vi "HB_SumStringOfBytes.vi"(1 "String Of Bytes":string) -> (0 "Sum as String":string)   [LabVIEW 2016]
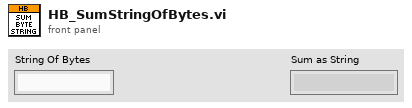
[diagram p1: front panel]
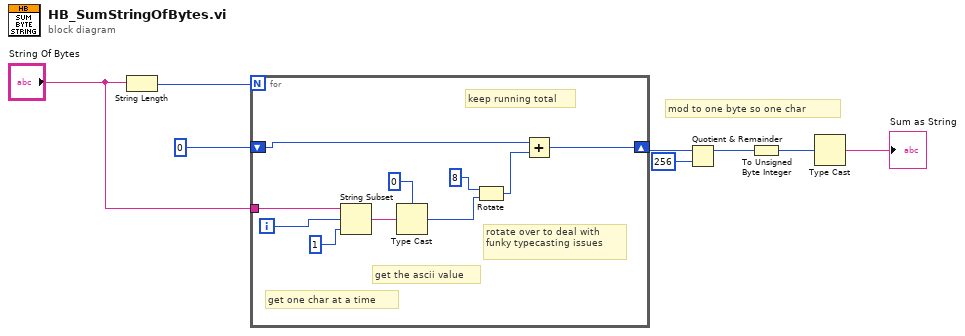
[diagram p0: block diagram]
diagram:
  # "mod to one byte so one char"
  n1 = String Length(string="String Of Bytes") -> (length=w8:i32)
  n2 = for {
    N: w8 -> [_]
    tunnel: "String Of Bytes" -> [w18]
    shift-right: [w12] -> w5
    shift-left: 0 -> [w13]
    i -> [w17]
    # "keep running total"
    # "rotate over to deal with\nfunky typecasting issues"
    # "get the ascii value"
    # "get one char at a time"
    n3 = String Subset(string=w18, offset (0)=w17, length (rest)=1 ("length (rest)")) -> (substring=w15:string)
    n4 = Type Cast(type=0 ("length (rest)"), x=w15) -> (*(type *) &x=w9:i32)
    n5 = Rotate(1:w9, 2:i16 8 ("y")) -> (0:w10:i32)
    n6 = Add(x=w13, y=w10) -> (x+y=w12:i32)
  }
  n7 = Quotient & Remainder(x=w5, y=256) -> (x-y*floor(x/y)=w2:i32)  [unwired: 1 out]
  n8 = To Unsigned Byte Integer(number=w2) -> (unsigned 8bit integer=w1:u8)
  n9 = Type Cast(x=w1) -> (*(type *) &x=→"Sum as String":string)  [unwired: 1 in]
